vi "fetchStimTrialStimulus.vi"(8 "error in (no error)":errorcluster, 11 "Stimulus in":refnum<class "Stimulus.lvclass">) -> (0 "error out":errorcluster, 2 "Stim":string, 3 "Stimulus out":refnum<class "Stimulus.lvclass">)   [LabVIEW 2014, in "Stimulus.lvclass"]
uses:
  Stimulus.lvclass
  Stimulus.lvclass/Stimulus.ctl
  <vilib>/vision/NI_Vision_Development_Module.lvlib
panel:
  out "logical OR":bool
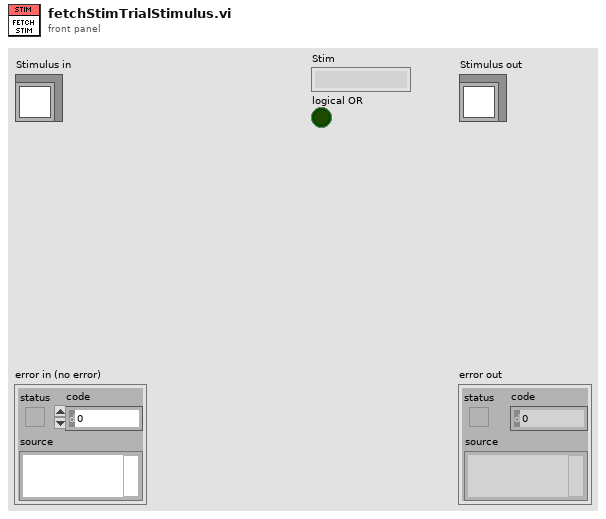
[diagram p1: front panel]
types:
  T1 = typedef "IMAQ Image.ctl" = refnum<image>
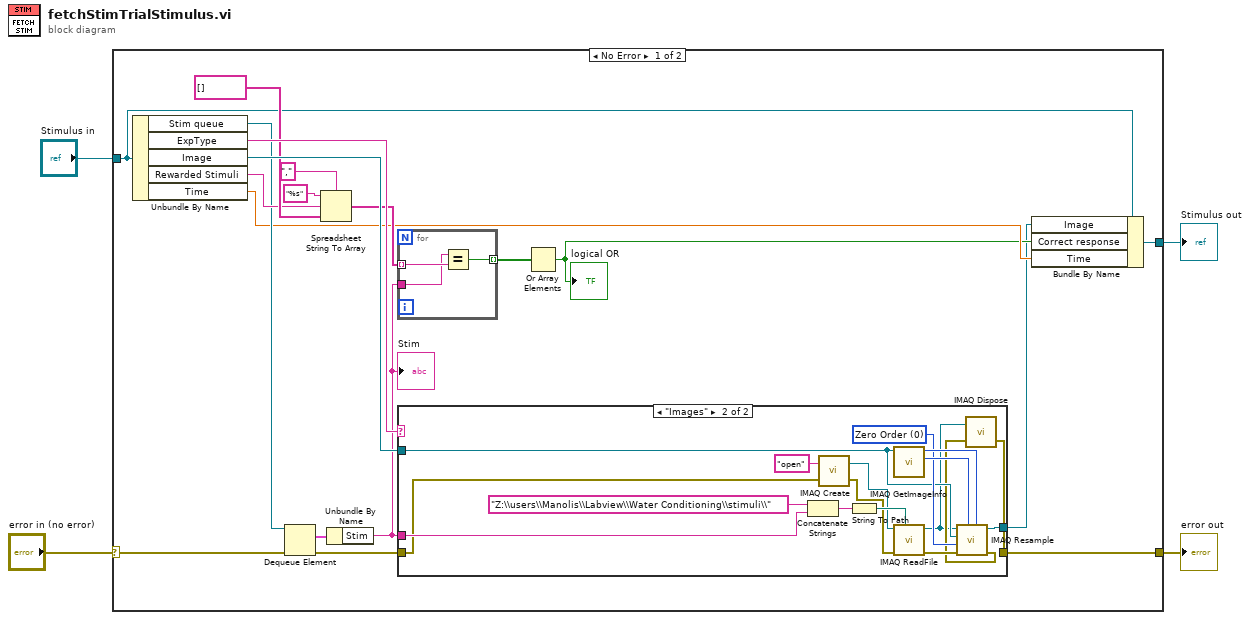
[diagram p0: block diagram]
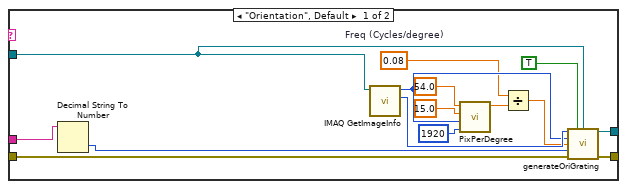
[diagram p2: hidden frame]
diagram:
  n1 = case shown="No Error" "error in (no error)" {
    selector: "error in (no error)" -> [w10 w60]
    tunnel: [w20 w60] -> w3
    tunnel: [w8 w59] -> w1
    tunnel: "Stimulus in" -> [w9 w59]
    frame No Error {
      n2 = Unbundle By Name(w9) -> ("Stim queue"=w11:refnum<queue>, "ExpType"=w23:string, "Image"=w19:T1, "Rewarded Stimuli"=w15:string, "Time"=w7:dbl)
      n3 = Dequeue Element(queue=w11, error in (no error)=w10) -> (element=w22:cluster{"Stim":string}, error out=w21:errorcluster)  [unwired: 1 in, 2 out]
      n4 = Spreadsheet String To Array(delimiter (Tab)=",", format string="%s", spreadsheet string=w15, array type (2D Dbl)=string[] []) -> (array=w13:string[])
      n5 = Unbundle By Name(w22) -> ("Stim"=w12:string)
      "Stim" <- w12
      n6 = for {
        tunnel: w13 -> [w26] mode=indexing
        tunnel: w12 -> [w25]
        tunnel: [w24] -> w14 mode=indexing
        n7 = Equal?(x=w25, y=w26) -> (x = y?=w24:bool)
      }
      n8 = case shown="\"Images\"" w23 {
        tunnel: w12 -> [w40 w56]
        tunnel: w21 -> [w38 w46]
        tunnel: [w37 w43] -> w20
        tunnel: w19 -> [w28 w49]
        tunnel: [w27 w54] -> w5
        frame "Orientation", Default {
          w30 = 0.08  # Freq (Cycles/degree)
          n9 = Decimal String To Number(string=w40) -> (number=w39:i32)  [unwired: 2 in, 1 out]
          n10 = call "IMAQ GetImageInfo"("Image"=w28) -> ("Y Resolution"=w36:i32, "X Resolution"=w35:i32)  [unwired: 3 in, 6 out]
          n11 = call "PixPerDegree.vi"("Monitor Resolution"=1920, "Resolution"=w35, "distance"=15.0, "Monitor Size"=54.0 ("Size")) -> ("Pixels/Degree"=w31:dbl)  [unwired: 6 in, 1 out]
          n12 = Divide(x=w30, y=w31) -> (x/y=w29:dbl)
          n13 = call "generateOriGrating.vi"("Y resolution"=w36, "Square?"=TRUE, "New Image"=w28, "X resolution"=w35, "frequency (cyc/pixel)"=w29, "Angle (degrees)"=w39, "error in (no error)"=w38) -> ("Image Dst Out"=w27:T1, "error out"=w37:errorcluster)  [unwired: 7 in]
        }
        frame "Images" {
          w50 = u32 0 items=["Zero Order", "Bi-Linear", "Quadratic", "Cubic Spline"] ("Interpolation Type")
          n14 = Concatenate Strings("Z:\\users\\Manolis\\Labview\\Water Conditioning\\stimuli\\" ("string"), w56) -> (w57:string)
          n15 = call "IMAQ Create"("Image Name"="open", "error in (no error)"=w46) -> ("New Image"=w47:T1, "error out"=w45:errorcluster)  [unwired: 3 in]
          n16 = String To Path(string=w57) -> (path=w58:path)
          n17 = call "IMAQ GetImageInfo"("Image"=w49) -> ("Y Resolution"=w52:i32, "X Resolution"=w51:i32)  [unwired: 3 in, 6 out]
          n18 = call "IMAQ ReadFile"("File Path"=w58, "error in (no error)"=w45, "Image"=w47) -> ("error out"=w53:errorcluster, "Image Out"=w42:T1)  [unwired: 4 in, 3 out]
          n19 = call "IMAQ Resample"("X Resolution"=w51, "Y Resolution"=w52, "error in (no error)"=w53, "Interpolation Type"=w50, "Image Dst"=w49, "Image Src"=w42) -> ("error out"=w44:errorcluster, "Image Dst Out"=w54:T1)  [unwired: 4 in]
          n20 = call "IMAQ Dispose"("Image"=w42, "error in (no error)"=w44) -> ("error out"=w43:errorcluster)  [unwired: 4 in]
        }
      }
      n21 = Or Array Elements(Boolean array=w14) -> (logical OR=w6:bool)
      "logical OR" <- w6
      n22 = Bundle By Name(cluster=w9, "Image"=w5, "Correct response"=w6, "Time"=w7) -> (w8:refnum<class "Stimulus.lvclass">)
    }
    frame Error {
    }
  }
  "error out" <- w3
  "Stimulus out" <- w1
